vi "Derivative x(t) (obs).vi"(2 "dt":dbl=1.0 format="%0.2f", 3 "final condition":dbl, 4 "initial condition":dbl, 5 "X":dbl[](array[numeric])) -> (0 "error":i32, 1 "dX/dt":dbl[](array[numeric]))   [LabVIEW 2017, in "NI_AALPro.lvlib"]
uses:
  NI_AALPro.lvlib
panel:
  # "This VI is obsolete !!!\nYou should replace this VI in your diagram with the Derivative x(t) VI.\n\nNOTE:   If you have wired to the initial condition and \n              final condition inputs of this obsolete VI, \n              please be aware that the new Derivative x(t) VI\n              accepts initial condition and finial condition \n              as array-based inputs."
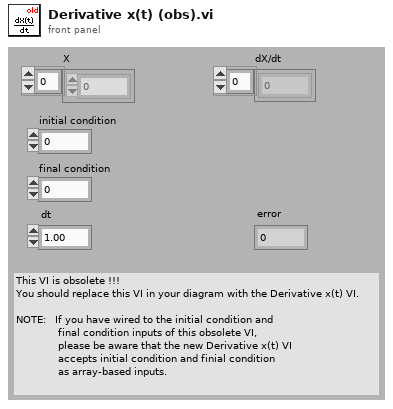
[diagram p1: front panel]
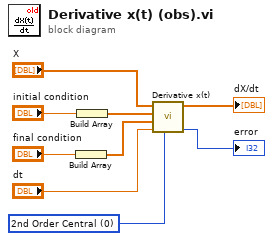
[diagram p0: block diagram]
diagram:
  w1 = u16 0 items=["2nd Order Central", "4th Order Central", "Forward", "Backward"] ("method")
  n1 = Build Array("final condition") -> (w3:dbl[])
  n2 = Build Array("initial condition") -> (w6:dbl[])
  n3 = call "Derivative x(t).vi"("method"=w1, "dt"="dt", "Final Condition"=w3, "Initial Condition"=w6, "X"="X") -> ("error"=→"error":i32, "dX/dt"=→"dX/dt":dbl[])  [unwired: 5 in]
